vi "Debug_Convert_Data_to_String.vi"(8 "error in (no error)":errorcluster, 11 "AB_Targetfile in":refnum<class "AB_Targetfile.lvclass">) -> (0 "error out":errorcluster, 2 "classData":string, 3 "AB_Targetfile out":refnum<class "AB_Targetfile.lvclass">)   [LabVIEW 2020, in "AB_Targetfile.lvclass"]
uses:
  <vilib>/AppBuilder/AB_Classes/TargetFile/AB_Targetfile.lvclass
  <vilib>/AppBuilder/AB_Classes/TargetFile/AB_Targetfile.lvclass/AB_Targetfile.ctl
  <vilib>/AppBuilder/AB_Classes/Build/AB_Build.lvclass
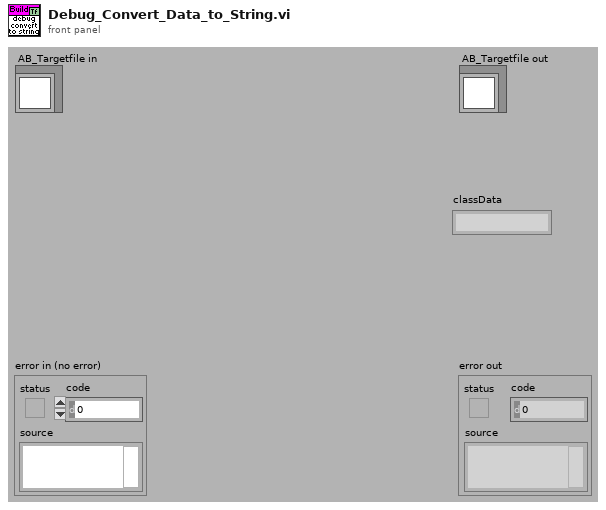
[diagram p1: front panel]
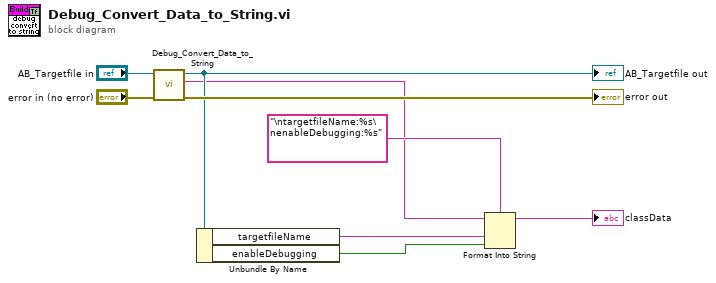
[diagram p0: block diagram]
diagram:
  n1 = call-parent "Debug_Convert_Data_to_String.vi"("error in (no error)"="error in (no error)", "AB_Build in"="AB_Targetfile in") -> ("error out"=→"error out":errorcluster, "classData"=w2:string, "AB_Build out"=w4:refnum<class "AB_Targetfile.lvclass">)  [unwired: 7 in]
  "AB_Targetfile out" <- w4
  n2 = Unbundle By Name(w4) -> ("targetfileName"=w5:string, "enableDebugging"=w3:bool)
  n3 = Format Into String(format string="\ntargetfileName:%s\nenableDebugging:%s", initial string=w2, w5, w3) -> (resulting string=→"classData":string)  [unwired: 1 in, 1 out]
